vi "AfterTest.vi"(0 "reference in":refnum<class "Test.lvclass">, 5 "error in (no error)":errorcluster) -> (14 "reference out":refnum<class "Test.lvclass">, 19 "error out":errorcluster)   [LabVIEW 2024, in "Test.lvclass"]
uses:
  Test.lvclass
  Test.lvclass/Test.ctl
panel:
  # "Connector Pane"
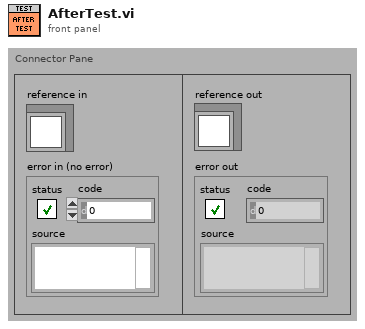
[diagram p1: front panel]
types:
  T1 = enum16{"Test Start", "Test Continue", "Test Failed", "Test Success"}
  T2 = typedef "Test.lvclass/ObjectAttributes.ctl" = cluster{"Engine":bool, "Dynamometer":bool, "Test Status":enum16{"Test Start", "Test Continue", "Test Failed", "Test Success"}, "History String":string}
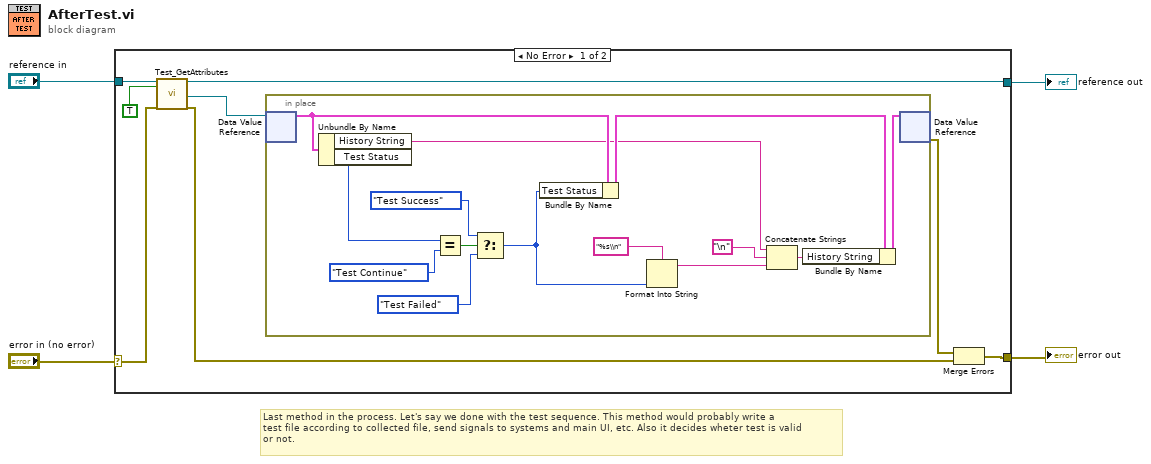
[diagram p0: block diagram]
diagram:
  # "Last method in the process. Let's say we done with the test sequence. This method would probably write a\ntest file according to collected file, send signals to systems and main UI, etc. Also it decides wheter test is valid\nor not."
  n1 = case shown="No Error" "error in (no error)" {
    selector: "error in (no error)" -> [w11 w28]
    tunnel: [w9 w28] -> w3
    tunnel: [w10 w27] -> w1
    tunnel: "reference in" -> [w12 w27]
    frame No Error {
      n2 = call "Test_GetAttributes.vi"("reference in"=w12, "OnlyGetDvrReference(False)"=TRUE, "error in (no error)"=w11) -> ("reference out"=w10:refnum<class "Test.lvclass">, "DataRef"=w6:refnum<data-value>, "error out"=w8:errorcluster)  [unwired: 13 in, 1 out]
      n3 = in-place {
        n4 = in-place-dvr #1(w6) -> (w25:T2)  [unwired: 1 out]
        n5 = Unbundle By Name(w25) -> ("History String"=w14:string, "Test Status"=w24:T1)
        n6 = Equal?(x=w24, y=T1."Test Continue") -> (x = y?=w22:bool)
        n7 = Select(t=T1."Test Success" ("y"), s=w22, f=T1."Test Failed" ("y")) -> (s? t:f=w19:T1)
        n8 = Bundle By Name(cluster=w25, "Test Status"=w19) -> (w26:T2)
        n9 = Format Into String(format string="%s\\n", w19) -> (resulting string=w16:string)  [unwired: 2 in, 1 out]
        n10 = Concatenate Strings(w14, "\n", w16) -> (w15:string)
        n11 = Bundle By Name(cluster=w26, "History String"=w15) -> (w17:T2)
        n12 = in-place-dvr #1(w17) -> (w5:errorcluster)  [unwired: 1 out]
      }
      n13 = Merge Errors(w5, w8) -> (w9:errorcluster)
    }
    frame Error {
    }
  }
  "error out" <- w3
  "reference out" <- w1
